vi "myRIO_BRig_FPGA_triggerLaserEvent.vi"(0 "I_laserEvent":bool, 1 "I_laser":bool, 2 "laser_selRew_Ntotal":u32=100, 3 "laser_selRew_Ndelay":u32, 4 "laser_selWro_Ntotal":u32=100, 5 "laser_selWro_NDelay":u32, 6 "counter":u32, 8 "I_startLaserEvent":bool, 9 "selectReward":bool, 10 "I_startLaser":bool) -> (12 "output_counter":u32, 14 "output_I_laserEvent":bool, 15 "output_I_laser":bool, 17 "output_I_trigLaserEvent":bool, 18 "output_I_trigLaser":bool)   [LabVIEW 2014]
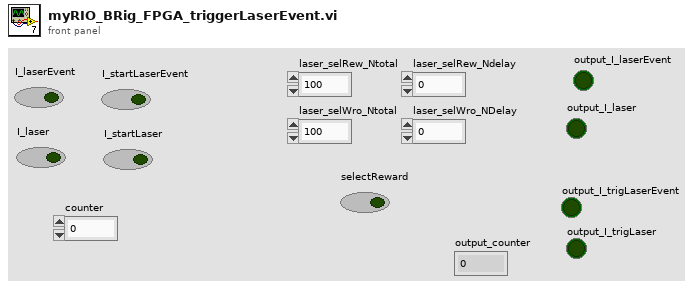
[diagram p1: front panel]
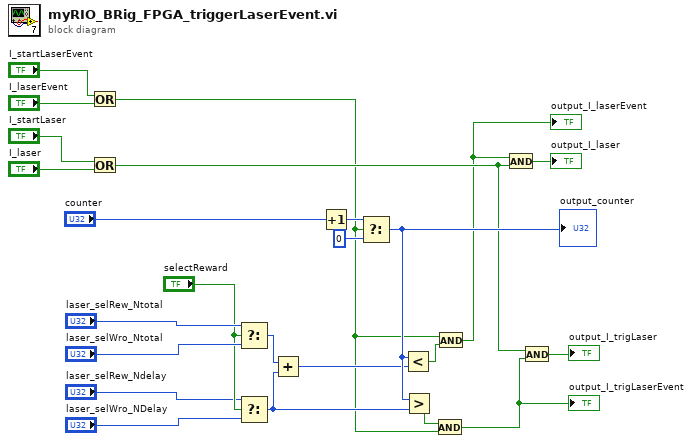
[diagram p0: block diagram]
diagram:
  n1 = Or(x="I_startLaserEvent", y="I_laserEvent") -> (x .or. y?=w2:bool)
  n2 = Or(x="I_startLaser", y="I_laser") -> (x .or. y?=w7:bool)
  n3 = Select(t="laser_selRew_Ntotal", s="selectReward", f="laser_selWro_Ntotal") -> (s? t:f=w12:u32)
  n4 = Select(t="laser_selRew_Ndelay", s="selectReward", f="laser_selWro_NDelay") -> (s? t:f=w9:u32)
  n5 = Add(x=w12, y=w9) -> (x+y=w10:u32)
  n6 = Increment(x="counter") -> (x+1=w15:u32)
  n7 = Select(t=w15, s=w2, f=u32 0) -> (s? t:f=w11:u32)
  "output_counter" <- w11
  n8 = Less?(x=w11, y=w10) -> (x < y?=w3:bool)
  n9 = Greater?(x=w11, y=w9) -> (0:w5:bool)
  n10 = And(x=w5, y=w2) -> (x .and. y?=w4:bool)
  "output_I_trigLaserEvent" <- w4
  n11 = And(x=w2, y=w3) -> (x .and. y?=w1:bool)
  "output_I_laserEvent" <- w1
  n12 = And(x=w1, y=w7) -> (x .and. y?=→"output_I_laser":bool)
  n13 = And(x=w7, y=w4) -> (x .and. y?=→"output_I_trigLaser":bool)
